vi "DriveWaitForBalls.vi"(2 "Parameter String":string, 3 "Reinit":bool) -> (0 "Error Out":errorcluster, 1 "Increment":bool)   [LabVIEW 2020]
doc: "This VI pauses the drive sequencer until the specified number of balls have been shot. It includes an option for a timeout.\n\nParameters:\n1. number of balls to be shot\n2. timeout (ms), or set to -1 to disable"
uses:
  SafeParser_Integer.vi
  drivercommands.vi
  sensordata.vi
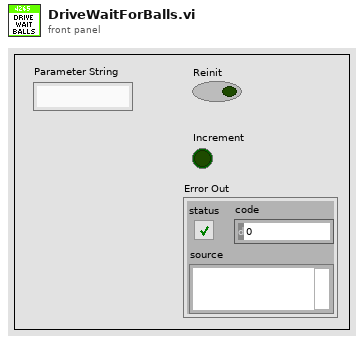
[diagram p1: front panel]
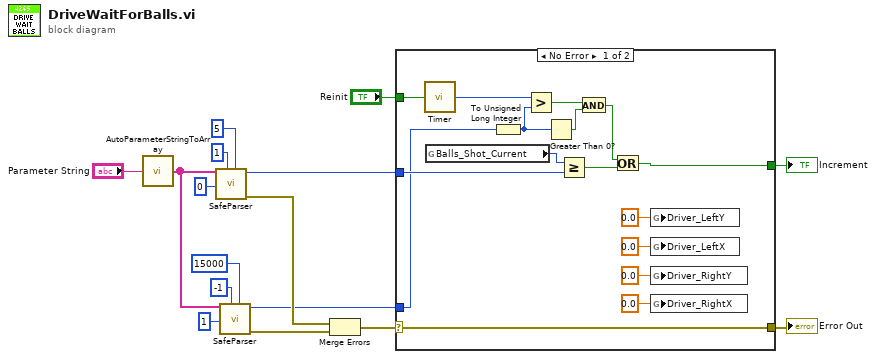
[diagram p0: block diagram]
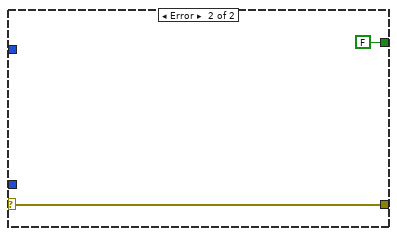
[diagram p2: hidden frame]
diagram:
  n1 = call "AutoParameterStringToArray.vi"("Parameter String"="Parameter String") -> ("Parsed Parameters"=w3:string[])
  n2 = call-poly "SafeParser.vi"("Maximum"=5, "Minimum"=1, "Array Index"=0 ("Parameter Index"), "String Array"=w3) -> ("Error Out"=w8:errorcluster, "Typecast  Value"=w12:i32)  [unwired: 6 in]
  n3 = call-poly "SafeParser.vi"("Maximum"=15000, "Minimum"=-1, "Array Index"=1 ("Parameter Index"), "String Array"=w3) -> ("Error Out"=w2:errorcluster, "Typecast  Value"=w1:i32)  [unwired: 6 in]
  n4 = Merge Errors(w8, w2) -> (w7:errorcluster)
  n5 = case shown="No Error" w7 {
    selector: w7 -> [w27 w34]
    tunnel: [w19 FALSE] -> w16
    tunnel: "Reinit" -> [w28 _]
    tunnel: [w27 w34] -> w14
    tunnel: w12 -> [w18 _]
    tunnel: w1 -> [w17 _]
    frame No Error {
      n6 = call "Timer.vi"("Reset Timer"=w28) -> ("Time (ms)"=w21:u32)
      n7 = global read "sensordata.vi" "Balls_Shot_Current"() -> (w26:i32)
      n8 = To Unsigned Long Integer(number=w17) -> (unsigned 32bit integer=w20:u32)
      n9 = Greater?(x=w21, y=w20) -> (0:w25:bool)
      n10 = Greater Than 0?(x=w20) -> (x > 0?=w24:bool)
      n11 = Greater Or Equal?(x=w26, y=w18) -> (x >= y?=w23:bool)
      n12 = And(x=w25, y=w24) -> (x .and. y?=w22:bool)
      n13 = Or(x=w22, y=w23) -> (x .or. y?=w19:bool)
      n14 = global write "drivercommands.vi" "Driver_LeftY"(0.0 ("Driver_LeftY")) -> ()
      n15 = global write "drivercommands.vi" "Driver_LeftX"(0.0 ("Driver_RightX")) -> ()
      n16 = global write "drivercommands.vi" "Driver_RightY"(0.0 ("Driver_RightX")) -> ()
      n17 = global write "drivercommands.vi" "Driver_RightX"(0.0 ("Driver_RightX")) -> ()
    }
    frame Error {
    }
  }
  "Increment" <- w16
  "Error Out" <- w14
